vi "SP Append Filter Limit Waveform.vi"(4 "Limit Format":T2, 5 "Number of Points":i32, 6 "Measured Parameter":T3={"Stimulus Port"=1, "Response Port"=1} {"Stimulus Port" min=1 step=1; "Response Port" min=1 step=1}, 7 "Attribute Name (NI_ChannelName)":string="NI_ChannelName", 8 "error in (no error)":errorcluster, 9 "Limits Pass/Fail":cluster{"Upper Pass?":bool, "Lower Pass?":bool}, 10 "Upper and Lower Limits":T1={"upper limit"={"x0"=0.0, "dx"=1.0, "Y"=[]}, "lower limit"={"x0"=0.0, "dx"=1.0, "Y"=[]}} {"lower limit"."Y" format="%.2p"; "lower limit"."dx" format="%.2p"; "lower limit"."x0" format="%.2p"; "upper limit"."Y" format="%.2p"; "upper limit"."dx" format="%.2p"; "upper limit"."x0" format="%.2p"}, 11 "Waveforms in":waveform(dbl)[](array[waveform])) -> (0 "error out":errorcluster, 3 "Waveforms out":waveform(dbl)[](array[waveform]))   [LabVIEW 2011]
uses:
  TypeDefs/SP Parameter.ctl
  TypeDefs/SP Format.ctl
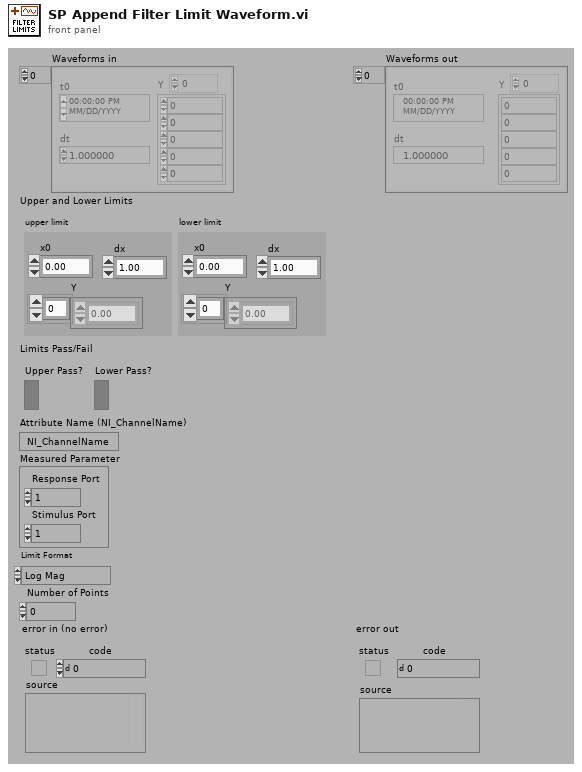
[diagram p1: front panel]
types:
  T1 = cluster{"upper limit":cluster{"x0":dbl, "dx":dbl, "Y":dbl[]}, "lower limit":cluster{"x0":dbl, "dx":dbl, "Y":dbl[]}}
  T2 = typedef "SP Format.ctl" = enum16{"Log Mag", "Lin Mag", "SWR", "Phase", "Expanded Phase", "Delay", "Insertion Loss", "Isolation", "Return Loss"}
  T3 = typedef "SP Parameter.ctl" = cluster{"Stimulus Port":i8, "Response Port":i8}
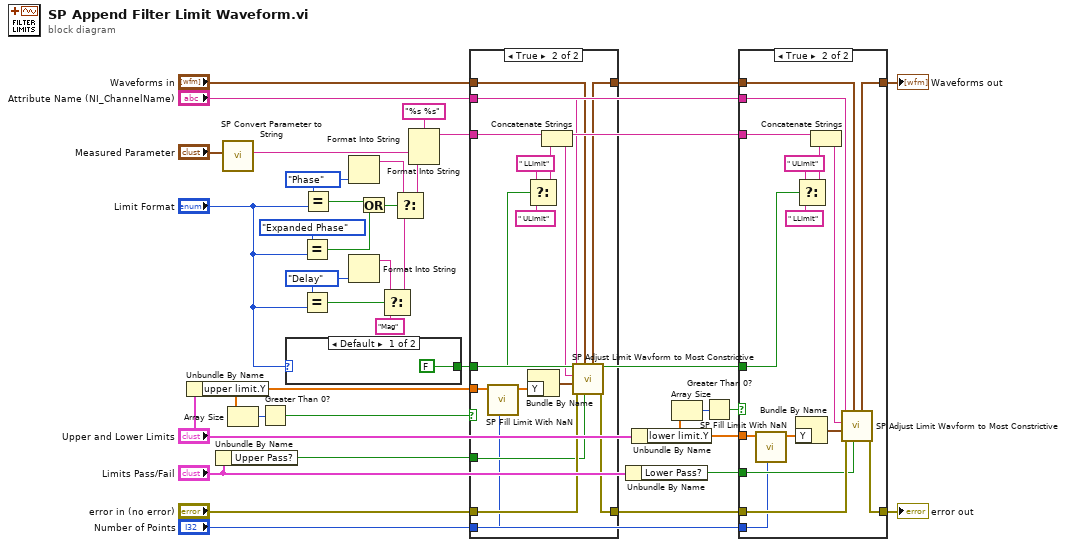
[diagram p0: block diagram]
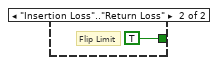
[diagram p2: hidden frame]
diagram:
  w25 = SP_Format."Delay" ("x")
  w28 = SP_Format."Phase" ("x")
  n1 = Unbundle By Name("Upper and Lower Limits") -> ("upper limit.Y"=w30:dbl[])
  n2 = Unbundle By Name("Limits Pass/Fail") -> ("Upper Pass?"=w20:bool)
  n3 = call "SP Convert Parameter to String.vi"("Parameter"="Measured Parameter") -> ("Parameter String"=w8:string)  [unwired: 10 out]
  n4 = Array Size(array=w30) -> (size(s)=w34:i32)
  n5 = Greater Than 0?(x=w34) -> (x > 0?=w31:bool)
  n6 = case shown="Default" "Limit Format" {
    tunnel: [FALSE TRUE] -> w7
    frame Default {
    }
    frame "Insertion Loss".."Return Loss" {
      # "Flip Limit"
    }
  }
  n7 = Equal?(x=SP_Format."Expanded Phase", y="Limit Format") -> (x = y?=w2:bool)
  n8 = Equal?(x=w25, y="Limit Format") -> (x = y?=w26:bool)
  n9 = Equal?(x=w28, y="Limit Format") -> (x = y?=w1:bool)
  n10 = Format Into String(w28) -> (resulting string=w27:string)  [unwired: 3 in, 1 out]
  n11 = Format Into String(w25) -> (resulting string=w24:string)  [unwired: 3 in, 1 out]
  n12 = Or(x=w1, y=w2) -> (x .or. y?=w5:bool)
  n13 = Select(t=w24, s=w26, f="Mag") -> (s? t:f=w23:string)
  n14 = Select(t=w27, s=w5, f=w23) -> (s? t:f=w32:string)
  n15 = Format Into String(format string="%s %s", w8, w32) -> (resulting string=w16:string)  [unwired: 2 in, 1 out]
  n16 = case shown="True" w31 {
    tunnel: "Waveforms in" -> [w39 w49]
    tunnel: "error in (no error)" -> [w40 w55]
    tunnel: [w40 w47] -> w13
    tunnel: "Attribute Name (NI_ChannelName)" -> [_ w45]
    tunnel: w30 -> [_ w43]
    tunnel: w16 -> [_ w54]
    tunnel: [w39 w48] -> w18
    tunnel: w20 -> [_ w46]
    tunnel: w7 -> [_ w50]
    tunnel: "Number of Points" -> [_ w41]
    frame False {
    }
    frame True {
      n17 = call "SP Fill Limit With NaN.vi"("Number of Points"=w41, "Limit"=w43) -> ("Filled Limit"=w42:dbl[])  [unwired: 9 out]
      n18 = Select(t=" LLimit", s=w50, f=" ULimit") -> (s? t:f=w51:string)
      n19 = Bundle By Name("Y"=w42) -> (w56:waveform(dbl))  [unwired: 1 out]
      n20 = Concatenate Strings(w54, w51) -> (w44:string)
      n21 = call "SP Adjust Limit Wavform to Most Constrictive.vi"("Pass?"=w46, "Waveforms In"=w49, "error in (no error)"=w55, "Waveform In"=w56, "Channel Name"=w44, "Attribute Name (NI_ChannelName)"=w45) -> ("error out"=w47:errorcluster, "Waveforms Out"=w48:waveform(dbl)[])  [unwired: 3 in, 1 out]
    }
  }
  n22 = Unbundle By Name("Limits Pass/Fail") -> ("Lower Pass?"=w12:bool)
  n23 = Unbundle By Name("Upper and Lower Limits") -> ("lower limit.Y"=w11:dbl[])
  n24 = Array Size(array=w11) -> (size(s)=w29:i32)
  n25 = Greater Than 0?(x=w29) -> (x > 0?=w10:bool)
  n26 = case shown="True" w10 {
    tunnel: w18 -> [w57 w66]
    tunnel: w13 -> [w58 w69]
    tunnel: [w58 w68] -> w14
    tunnel: "Attribute Name (NI_ChannelName)" -> [_ w65]
    tunnel: w11 -> [_ w61]
    tunnel: w16 -> [_ w74]
    tunnel: [w57 w67] -> w15
    tunnel: w12 -> [_ w62]
    tunnel: w7 -> [_ w70]
    tunnel: "Number of Points" -> [_ w59]
    frame False {
    }
    frame True {
      n27 = call "SP Fill Limit With NaN.vi"("Number of Points"=w59, "Limit"=w61) -> ("Filled Limit"=w60:dbl[])  [unwired: 9 out]
      n28 = Bundle By Name("Y"=w60) -> (w63:waveform(dbl))  [unwired: 1 out]
      n29 = Select(t=" ULimit", s=w70, f=" LLimit") -> (s? t:f=w71:string)
      n30 = Concatenate Strings(w74, w71) -> (w64:string)
      n31 = call "SP Adjust Limit Wavform to Most Constrictive.vi"("Pass?"=w62, "Waveforms In"=w66, "error in (no error)"=w69, "Waveform In"=w63, "Channel Name"=w64, "Attribute Name (NI_ChannelName)"=w65) -> ("error out"=w68:errorcluster, "Waveforms Out"=w67:waveform(dbl)[])  [unwired: 3 in, 1 out]
    }
  }
  "Waveforms out" <- w15
  "error out" <- w14
